vi "optimize swerve.vi"(8 "error in (no error)":errorcluster, 9 "current angle (deg)":dbl=5.0, 10 "target angle (deg)":dbl, 11 "velocity":dbl) -> (0 "error out":errorcluster, 1 "reset POS to ABS":bool, 2 "steer angle (deg)":dbl=90.0, 3 "velocity":dbl)   [LabVIEW 2023]
uses:
  <vilib>/Analysis/coordinate.llb/Angle Units.ctl
  <vilib>/Analysis/coordinate.llb/Angle Range (Degree).ctl
  <vilib>/Analysis/coordinate.llb/Wrap Angle (scalar).vi
  <vilib>/Analysis/NI_AAL_Angle.lvlib
panel:
  in  "deadband\nvelocity":dbl=0.025 format="%#_13g"
  in  "@rest streering angle":dbl=90.0
  out "min index(es)":i32
  out "delta\noptions":dbl[](array[numeric])=[85.0, 445.0, -275.0, 265.0, -95.0]
  out "invert V":bool
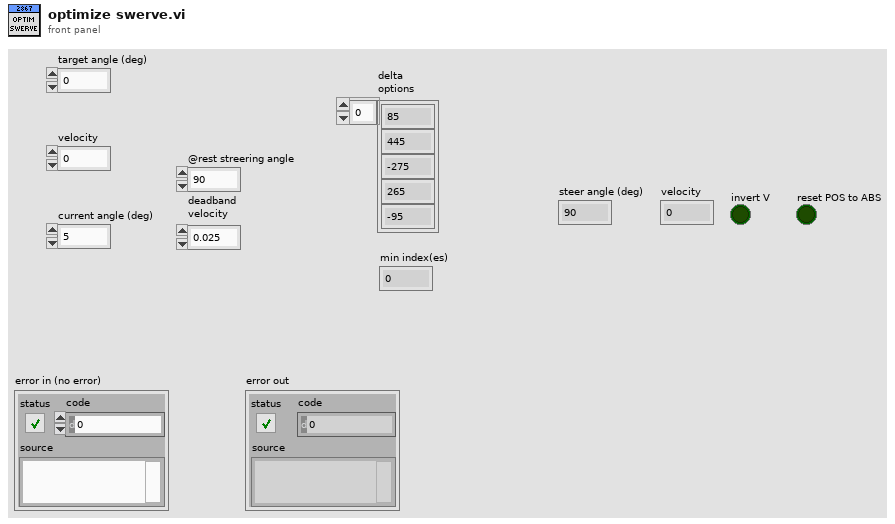
[diagram p1: front panel]
types:
  T1 = typedef "NI_AAL_Angle.lvlib/Angle Range (Degree).ctl" = u16
  T2 = typedef "NI_AAL_Angle.lvlib/Angle Units.ctl" = i32
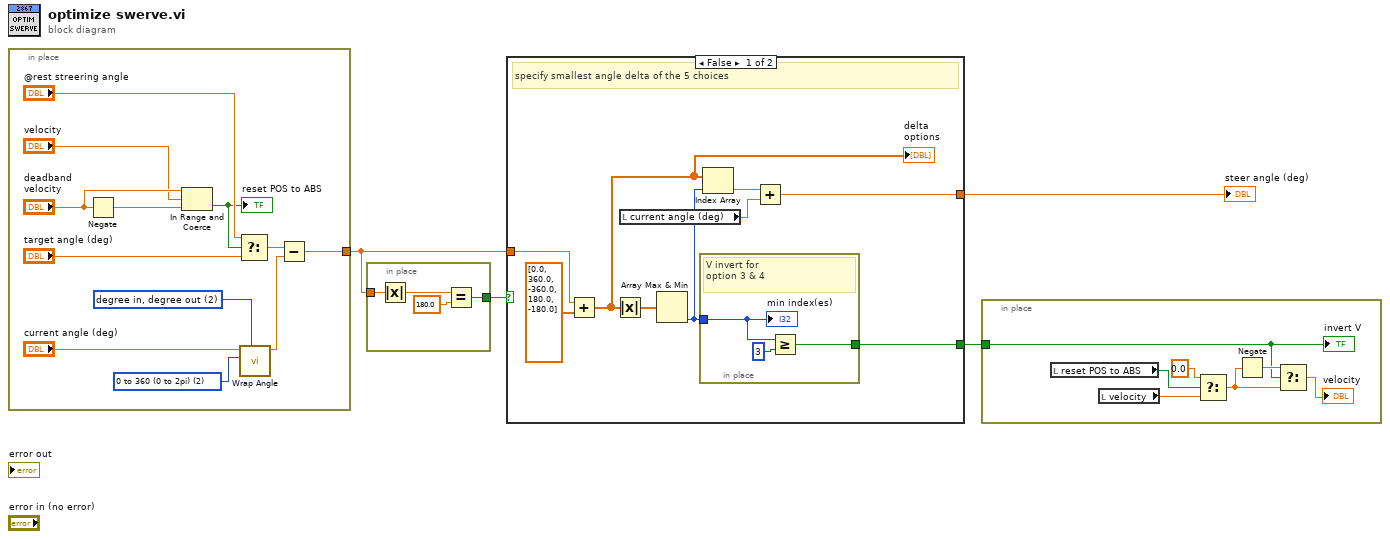
[diagram p0: block diagram]
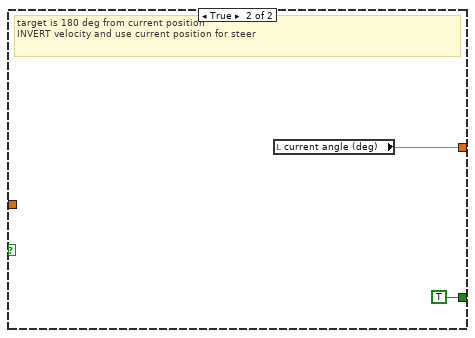
[diagram p2: hidden frame]
diagram:
  n1 = in-place {
    in-place-border: [w6] -> w1
    w15 = T1 2 items=["none", "-180 to 180 (-pi to pi)", "0 to 360 (0 to 2pi)"] ("angle range")
    w16 = T2 2 items=["radian in, radian out", "radian in, degree out", "degree in, degree out", "degree in, radian out"] ("angle units")
    n2 = Negate(x="deadband\nvelocity") -> (-x=w9:dbl)
    n3 = In Range and Coerce(upper limit="deadband\nvelocity", x="velocity", lower limit=w9) -> (In Range?=w7:bool)  [unwired: 1 out]
    "reset POS to ABS" <- w7
    n4 = Select(t="@rest streering angle", s=w7, f="target angle (deg)") -> (s? t:f=w11:dbl)
    n5 = call-poly <vilib>:"Wrap Angle.vi"("angle units"=w16, "angle range"=w15, "angle in"="current angle (deg)") -> ("angle out"=w12:dbl)  [unwired: 7 in, 1 out]
    n6 = Subtract(x=w11, y=w12) -> (x-y=w6:dbl)
  }
  n7 = in-place {
    in-place-border: [w20] -> w2
    in-place-border: w1 -> [w18]
    n8 = Absolute Value(x=w18) -> (abs(x)=w17:dbl)
    n9 = Equal?(x=w17, y=180.0) -> (x = y?=w20:bool)
  }
  n10 = case shown="False" w2 {
    tunnel: w1 -> [w28 _]
    tunnel: [w22 w34] -> w4
    tunnel: [w23 TRUE] -> w3
    frame False {
      # "specify smallest angle delta of the 5 choices"
      n11 = Add(x=w28, y=dbl[] [0.0, 360.0, -360.0, 180.0, -180.0]) -> (x+y=w26:dbl[])
      "delta\noptions" <- w26
      n12 = Absolute Value(x=w26) -> (abs(x)=w27:dbl[])
      n13 = local read "current angle (deg)"() -> (w21:dbl)
      n14 = Array Max & Min(array=w27) -> (min index (indices)=w24:i32)  [unwired: 3 out]
      n15 = in-place {
        in-place-border: w24 -> [w30]
        in-place-border: [w31] -> w23
        # "V invert for \noption 3 & 4"
        n16 = Greater Or Equal?(x=w30, y=3) -> (x >= y?=w31:bool)
        "min index(es)" <- w30
      }
      n17 = Index Array(array=w26, index=w24) -> (element=w25:dbl)
      n18 = Add(x=w25, y=w21) -> (x+y=w22:dbl)
    }
    frame True {
      # "target is 180 deg from current position\nINVERT velocity and use current position for steer"
      n19 = local read "current angle (deg)"() -> (w34:dbl)
    }
  }
  "steer angle (deg)" <- w4
  n20 = in-place {
    in-place-border: w3 -> [w39]
    n21 = local read "reset POS to ABS"() -> (w36:bool)
    n22 = local read "velocity"() -> (w37:dbl)
    n23 = Select(t=0.0, s=w36, f=w37) -> (s? t:f=w38:dbl)
    n24 = Negate(x=w38) -> (-x=w40:dbl)
    n25 = Select(t=w40, s=w39, f=w38) -> (s? t:f=→"velocity":dbl)
    "invert V" <- w39
  }
